vi "Init.vi"(8 "error in (no error)":errorcluster, 10 "Scene Item ID":i32, 11 "Scene Name":string) -> (0 "error out":errorcluster, 3 "GetSceneItemTransform out":refnum<class "GetSceneItemTransform.lvclass">)   [LabVIEW 2020, in "obs-websocket.lvlib" / "GetSceneItemTransform.lvclass"]
uses:
  GetSceneItemTransform.lvclass
  GetSceneItemTransform.lvclass/GetSceneItemTransform.ctl
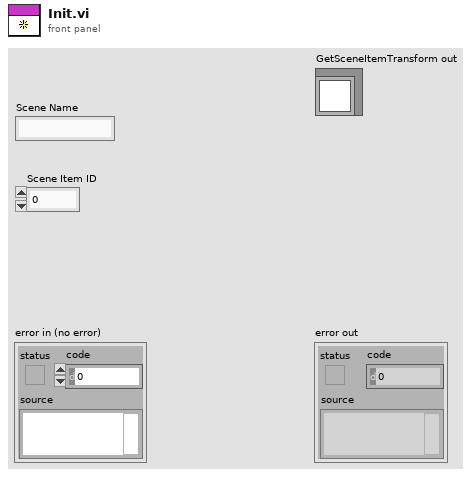
[diagram p1: front panel]
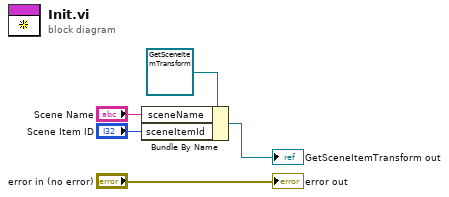
[diagram p0: block diagram]
diagram:
  n1 = Bundle By Name(cluster=refnum<class "GetSceneItemTransform.lvclass"> refnum ("GetSceneItemTransform in"), "sceneName"="Scene Name", "sceneItemId"="Scene Item ID") -> (→"GetSceneItemTransform out":refnum<class "GetSceneItemTransform.lvclass">)
  "error out" <- "error in (no error)"
